vi "get thread pool.vi"(11 "task in":refnum<class "task.lvclass">) -> (2 "dispatcher":refnum<data-value>, 3 "task out":refnum<class "task.lvclass">)   [LabVIEW 2013, in "task.lvclass"]
uses:
  task.lvclass
  dispatcher/thread pool.lvclass
  task.lvclass/task.ctl
  dispatcher/dispatcher api type.ctl
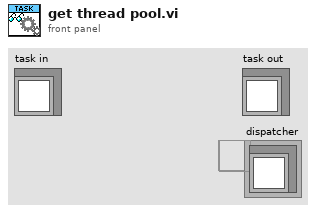
[diagram p1: front panel]
types:
  T1 = typedef "thread pool.lvclass/dispatcher api type.ctl" = refnum<data-value>
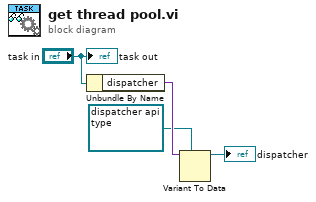
[diagram p0: block diagram]
diagram:
  n1 = Unbundle By Name("task in") -> ("dispatcher"=w3:variant)
  n2 = Variant To Data(type=T1 refnum ("dispatcher"), Variant=w3) -> (data=→"dispatcher":T1)  [unwired: 1 in, 1 out]
  "task out" <- "task in"
